vi "move.vi"(2 "func":i32, 3 "ID":i32, 4 "handle":i32, 5 "错误输入（无错误）":errorcluster) -> (0 "return":i32, 1 "错误输出":errorcluster)   [LabVIEW 2013, in "EM_CVx.lvlib"]
uses:
  EM_CVx.lvlib
  library/moverLibrary_x86.dll
  library/moverLibrary_x64.dll
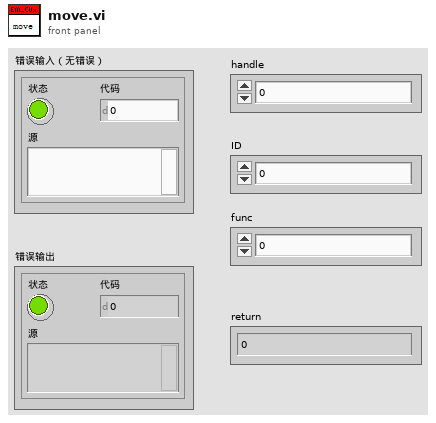
[diagram p1: front panel]
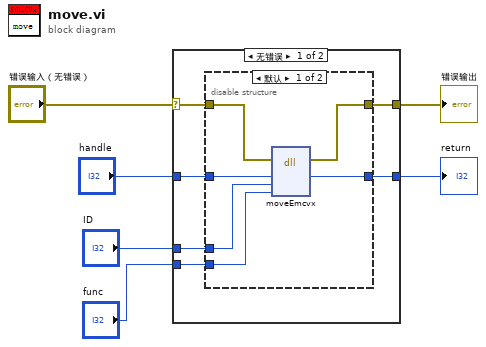
[diagram p0: block diagram]
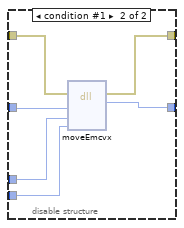
[diagram p2: hidden frame]
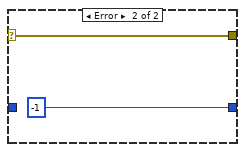
[diagram p3: hidden frame]
diagram:
  n1 = case shown="无错误" "错误输入（无错误）" {
    selector: "错误输入（无错误）" -> [w12 w26]
    tunnel: [w11 w26] -> w5
    tunnel: [w10 -1 ("return")] -> w4
    tunnel: "handle" -> [w9 _]
    tunnel: "ID" -> [w8 _]
    tunnel: "func" -> [w7 _]
    frame No Error {
      n2 = disable-structure shown="默认" {
        disable-tunnel: w12 -> [w18 w24]
        disable-tunnel: [w17 w23] -> w11
        disable-tunnel: [w16 w19] -> w10
        disable-tunnel: w9 -> [w15 w22]
        disable-tunnel: w8 -> [w14 w21]
        disable-tunnel: w7 -> [w13 w20]
        frame condition #0 (active) {
          n3 = dll-call lib="E:/5-mover/4-labView/EM_CVx_2013/library/moverLibrary_x86.dll" fn="moveEmcvx"(error in=w18, "handle"=w15, "ID"=w14, "func"=w13) -> (error out=w17:errorcluster, "return"=w16:i32)  [unwired: 5 in, 1 out]
        }
        frame condition #1 {
          n4 = dll-call lib="E:/5-mover/4-labView/EM_CVx_2013/library/moverLibrary_x64.dll" fn="moveEmcvx"(error in=w24, "handle"=w22, "ID"=w21, "func"=w20) -> (error out=w23:errorcluster, "return"=w19:i32)  [unwired: 5 in, 1 out]
        }
      }
    }
    frame Error {
    }
  }
  "错误输出" <- w5
  "return" <- w4
